vi "Mouse Click.vi"(8 "error in (no error)":errorcluster, 9 "ms wait after up (10)":u32=10, 10 "ms wait after down (10)":u32=10, 11 "Right Click? (F)":bool) -> (0 "error out":errorcluster)   [LabVIEW 2017]
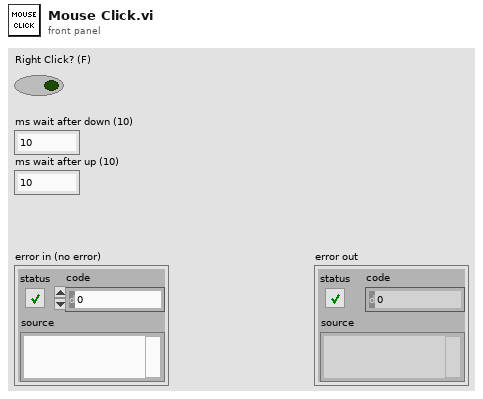
[diagram p1: front panel]
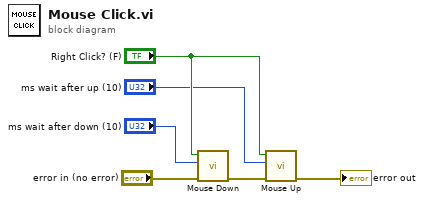
[diagram p0: block diagram]
diagram:
  n1 = call "Mouse Down.vi"("error in (no error)"="error in (no error)", "Delay in ms (10)"="ms wait after down (10)", "Right Click? (F)"="Right Click? (F)") -> ("error out"=w3:errorcluster)  [unwired: 8 in]
  n2 = call "Mouse Up.vi"("error in (no error)"=w3, "Delay in ms (10)"="ms wait after up (10)", "Right Click? (F)"="Right Click? (F)") -> ("error out"=→"error out":errorcluster)  [unwired: 8 in]
